vi "unflat.vi"(5 "Numeric":u32) -> (2 "*(type *) &x":refnum<k5>)   [LabVIEW 2012]
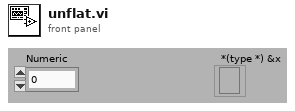
[diagram p1: front panel]
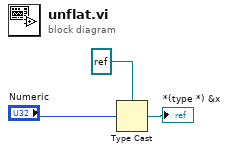
[diagram p0: block diagram]
diagram:
  n1 = Type Cast(type=refnum<k5> refnum ("connection ID"), x="Numeric") -> (*(type *) &x=→"*(type *) &x":refnum<k5>)
